vi "ReadLimits.vi"(0 "Interface in":T1, 11 "error in (no error)":errorcluster) -> (4 "Interface out":T1, 6 "Limits":string, 15 "error out":errorcluster)   [LabVIEW 2017, in "ScaleAndLimitInterface.lvlib"]
doc: "Read the limits registers and translate to a string that indications which limits are tripped."
uses:
  ScaleAndLimitInterface.lvlib
  Interface.ctl
  <instrlib>/_niInstr/Instruction Framework/v1/Host/Instruction Framework Context/niInstr Instruction Framework Context v1 Host.lvclass
  <instrlib>/_niInstr/Instruction Framework/v1/Host/Instruction Target/niInstr Instruction Target v1 Host.lvclass
  Configuration.ctl
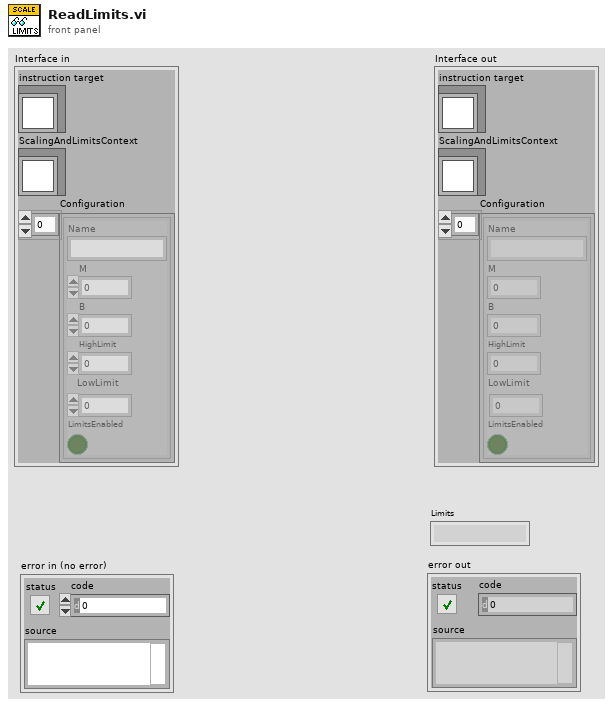
[diagram p1: front panel]
types:
  T1 = typedef "ScaleAndLimitInterface.lvlib/Interface.ctl" = cluster{"instruction target":refnum<class "niInstr Instruction Target v1 Host.lvclass">, "ScalingAndLimitsContext":refnum<class "niInstr Instruction Framework Context v1 Host.lvclass">, "Configuration":T2[]}
  T2 = typedef "ScaleAndLimitInterface.lvlib/Configuration.ctl" = cluster{"Name":string, "M":dbl, "B":i16, "HighLimit":dbl, "LowLimit":dbl, "LimitsEnabled":bool}
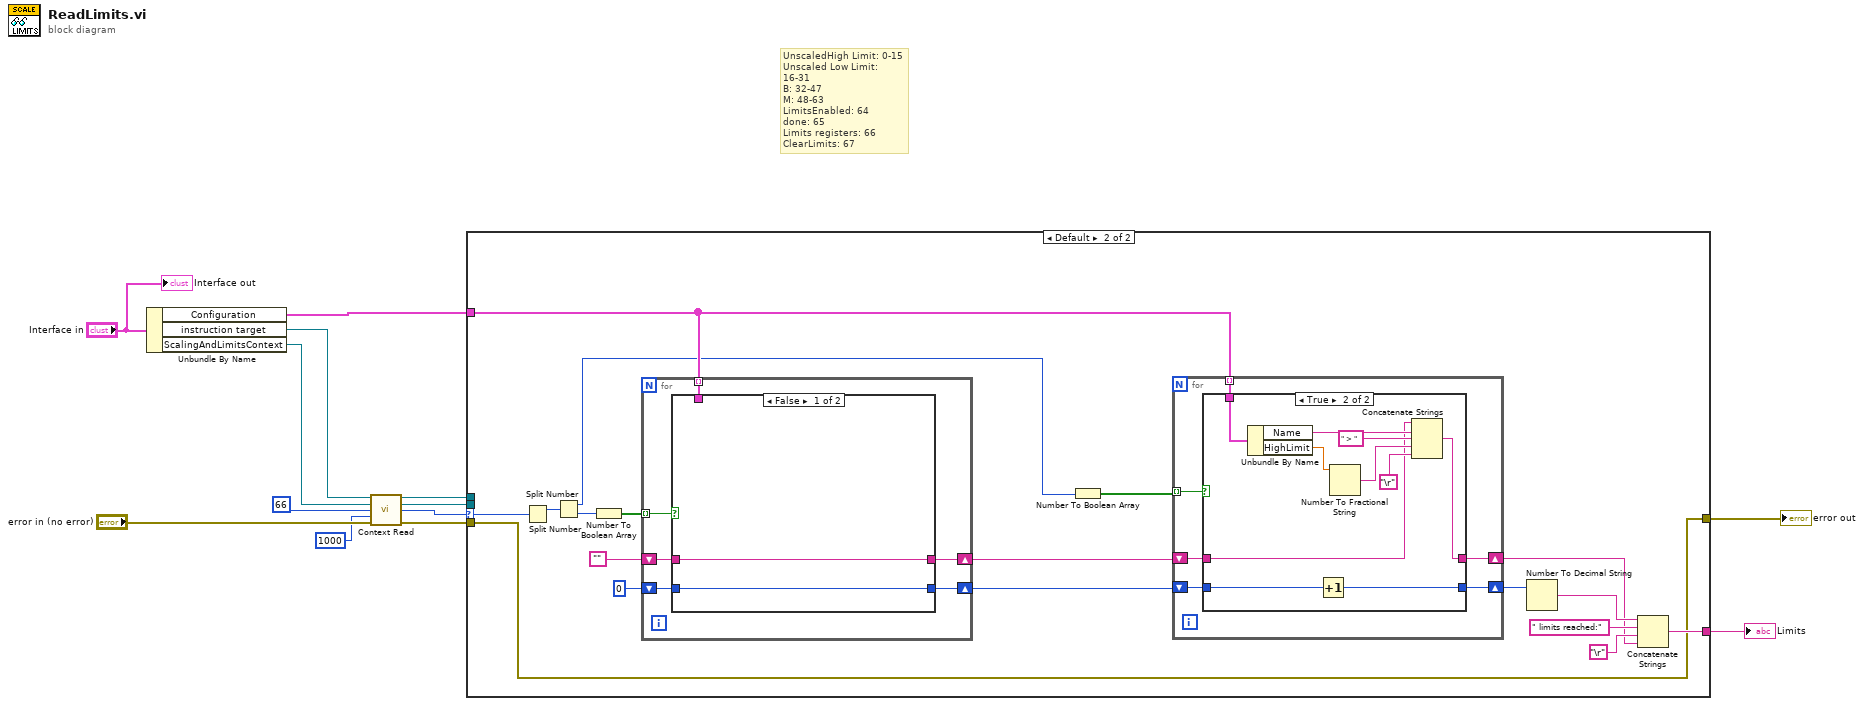
[diagram p0: block diagram]
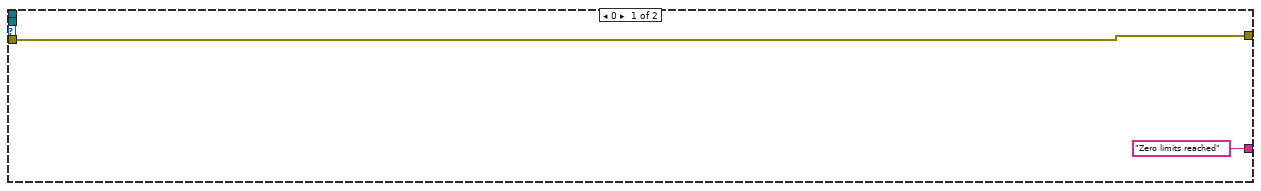
[diagram p2: hidden frame]
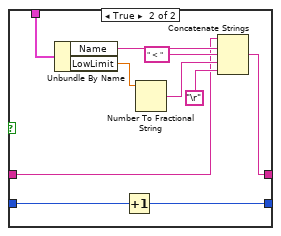
[diagram p4: hidden frame]
diagram:
  # "UnscaledHigh Limit: 0-15\nUnscaled Low Limit: 16-31\nB: 32-47\nM: 48-63\nLimitsEnabled: 64\ndone: 65\nLimits registers: 66\nClearLimits: 67"
  n1 = Unbundle By Name("Interface in") -> ("Configuration"=w10:T2[], "instruction target"=w7:refnum<class "niInstr Instruction Target v1 Host.lvclass">, "ScalingAndLimitsContext"=w6:refnum<class "niInstr Instruction Framework Context v1 Host.lvclass">)
  n2 = call <instrlib>:"Context Read.vi"("instruction target in"=w7, "context in"=w6, "address"=u64 66, "timeout (5000 ms)"=1000, "error in"="error in (no error)") -> ("instruction target out"=w2:refnum<class "niInstr Instruction Target v1 Host.lvclass">, "context out"=w1:refnum<class "niInstr Instruction Framework Context v1 Host.lvclass">, "data"=w3:u64, "error out"=w8:errorcluster)  [unwired: 7 in]
  n3 = case shown="Default" w3 {
    selector: w3 -> [_ w20]
    tunnel: w8 -> [w15 w16]
    tunnel: w10 -> [_ w30]
    tunnel: [w15 w16] -> w13
    tunnel: ["Zero limits reached" w21] -> w12
    tunnel: w2 -> [_ _]
    tunnel: w1 -> [_ _]
    frame 0 {
    }
    frame Default {
      n4 = Split Number(x=w20) -> (hi(x)=w19:u32)  [unwired: 1 out]
      n5 = Split Number(x=w19) -> (hi(x)=w17:u16, lo(x)=w18:u16)
      n6 = Number To Boolean Array(number=w18) -> (Boolean array=w33:bool[])
      n7 = for {
        tunnel: w30 -> [w54] mode=indexing
        tunnel: w33 -> [w57] mode=indexing
        shift-right: [w55] -> w27
        shift-left: "" -> [w56]
        shift-right: [w52] -> w28
        shift-left: 0 -> [w53]
        n8 = case shown="False" w57 {
          tunnel: w56 -> [w59 w61]
          tunnel: [w59 w60] -> w55
          tunnel: w54 -> [_ w69]
          tunnel: w53 -> [w58 w68]
          tunnel: [w58 w67] -> w52
          frame False {
          }
          frame True {
            n9 = Unbundle By Name(w69) -> ("Name"=w66:string, "LowLimit"=w64:dbl)
            n10 = Increment(x=w68) -> (x+1=w67:i32)
            n11 = Number To Fractional String(number=w64) -> (F-format string=w63:string)  [unwired: 3 in]
            n12 = Concatenate Strings(w61, w66, " < " ("string"), w63, "\r") -> (w60:string)
          }
        }
      }
      n13 = Number To Boolean Array(number=w17) -> (Boolean array=w29:bool[])
      n14 = for {
        tunnel: w30 -> [w36] mode=indexing
        tunnel: w29 -> [w39] mode=indexing
        shift-right: [w37] -> w22
        shift-left: w27 -> [w38]
        shift-right: [w34] -> w26
        shift-left: w28 -> [w35]
        n15 = case shown="True" w39 {
          tunnel: w38 -> [w41 w43]
          tunnel: [w41 w42] -> w37
          tunnel: w36 -> [_ w51]
          tunnel: w35 -> [w40 w50]
          tunnel: [w40 w49] -> w34
          frame False {
          }
          frame True {
            n16 = Unbundle By Name(w51) -> ("Name"=w48:string, "HighLimit"=w46:dbl)
            n17 = Increment(x=w50) -> (x+1=w49:i32)
            n18 = Number To Fractional String(number=w46) -> (F-format string=w45:string)  [unwired: 3 in]
            n19 = Concatenate Strings(w43, w48, " > " ("string"), w45, "\r") -> (w42:string)
          }
        }
      }
      n20 = Number To Decimal String(number=w26) -> (decimal integer string=w24:string)  [unwired: 1 in]
      n21 = Concatenate Strings(w24, " limits reached:" ("string"), "\r", w22) -> (w21:string)
    }
  }
  "error out" <- w13
  "Limits" <- w12
  "Interface out" <- "Interface in"
